vi "Drive_Global.vi"() -> ()   [LabVIEW 2015]
panel:
  in  "Auto_Far_Shoot":bool
  in  "Completed_Auto":bool
  in  "Cam_New_Image":bool
  in  "Auto_Stage":bool
  in  "Auto_Shoot":bool
  in  "Auto_Intake_Arm_Lower":bool
  out "Vision Distance":cluster{"1":dbl, "2":dbl, "3":dbl}
  in  "Aimed?":bool
  in  "Lower_Arms":bool
  in  "Reset_Encoder":bool
  in  "Comp_Robot?":bool
  in  "Enable_Cam":bool
  out "Vision_angle":cluster{"1":dbl, "2":dbl, "3":dbl}
  in  "Wheel Speed":dbl
  in  "High_Gear":bool
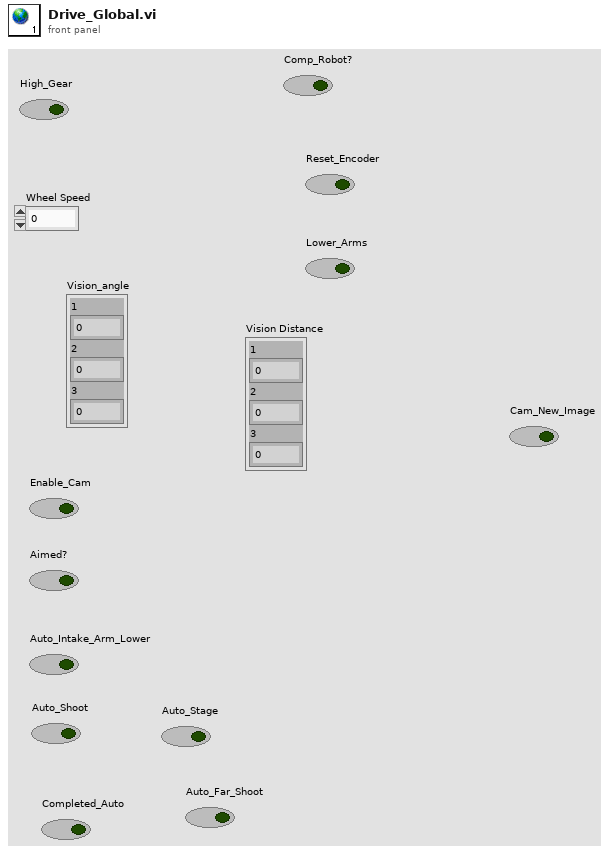
[diagram p1: front panel]
diagram:
